vi "greaterlessequal.vi"(10 "y":dbl format="%.2f", 11 "x":dbl format="%.2f") -> (7 "comparison":enum16{"less than", "equal to", "greater than"}(ring))   [LabVIEW 2012]
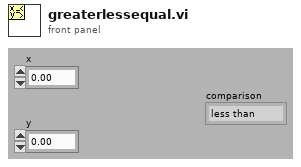
[diagram p1: front panel]
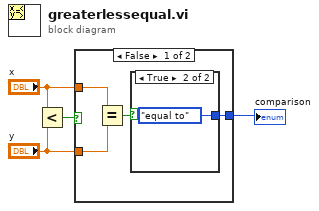
[diagram p0: block diagram]
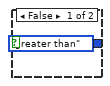
[diagram p2: hidden frame]
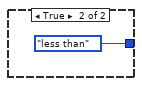
[diagram p3: hidden frame]
diagram:
  n1 = Less?(x="x", y="y") -> (x < y?=w4:bool)
  n2 = case shown="False" w4 {
    tunnel: [w5 enum16{"less than", "equal to", "greater than"}."less than" ("comparison")] -> w3
    tunnel: "y" -> [w8 _]
    tunnel: "x" -> [w7 _]
    frame False {
      n3 = Equal?(x=w7, y=w8) -> (x = y?=w6:bool)
      n4 = case shown="True" w6 {
        tunnel: [enum16{"less than", "equal to", "greater than"}."greater than" ("comparison") enum16{"less than", "equal to", "greater than"}."equal to" ("comparison")] -> w5
        frame False {
        }
        frame True {
        }
      }
    }
    frame True {
    }
  }
  "comparison" <- w3
